vi "FetchCalibration.vi"(8 "error in (no error)":errorcluster, 10 "instruments":string[](array[string]), 11 "ByteGSAPIBase in":refnum<class "ByteGSAPIBase.lvclass">) -> (0 "error out":errorcluster, 2 "instruments":T1[](array[typedef]), 3 "ByteGSAPIBase out":refnum<class "ByteGSAPIBase.lvclass">)   [LabVIEW 2019, in "ByteGSWebAPI.lvlib" / "ByteGSAPIBase.lvclass"]
doc: "Obtain instruments calibrations based on the Instrument Slug"
uses:
  ByteGSAPIBase.lvclass
  Converted_Slug_Cluster.ctl
  <vilib>/Bytelabs/ByteREST/ByteRESTClass/ByteRESTBase/HTTP/Status_Code.ctl
  JSON_Slug_Cluster.ctl
  ByteGSAPIBase.lvclass/ByteGSAPIBase.ctl
  <vilib>/Bytelabs/ByteREST/ByteRESTClass/ByteRESTBase/RESTBase.lvclass
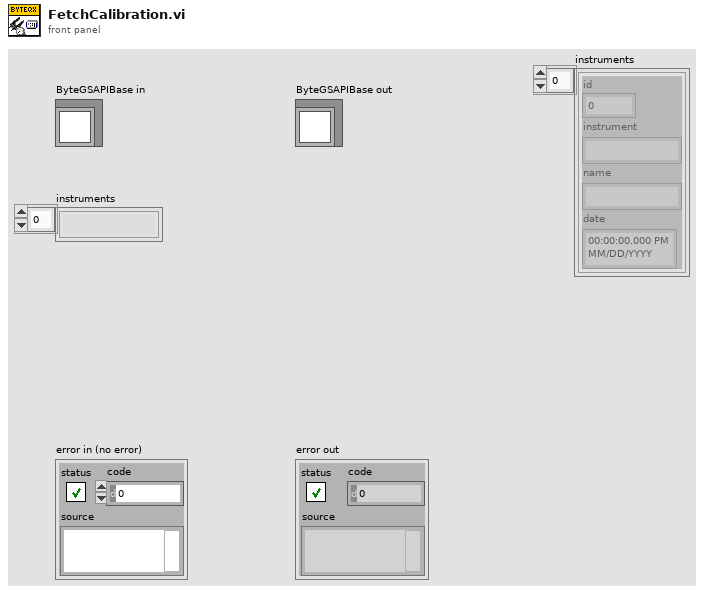
[diagram p1: front panel]
types:
  T1 = typedef "ByteGSWebAPI.lvlib/ByteGSAPIBase.lvclass/Converted_Slug_Cluster.ctl" = cluster{"id":u32, "instrument":string, "name":string, "date":timestamp}
  T2 = typedef "ByteGSWebAPI.lvlib/ByteGSAPIBase.lvclass/JSON_Slug_Cluster.ctl" = cluster{"id":u32, "instrument":string, "name":string, "data":string}
  T3 = typedef "ByteREST.lvlib/RESTBase.lvclass/Status_Code.ctl" = u16
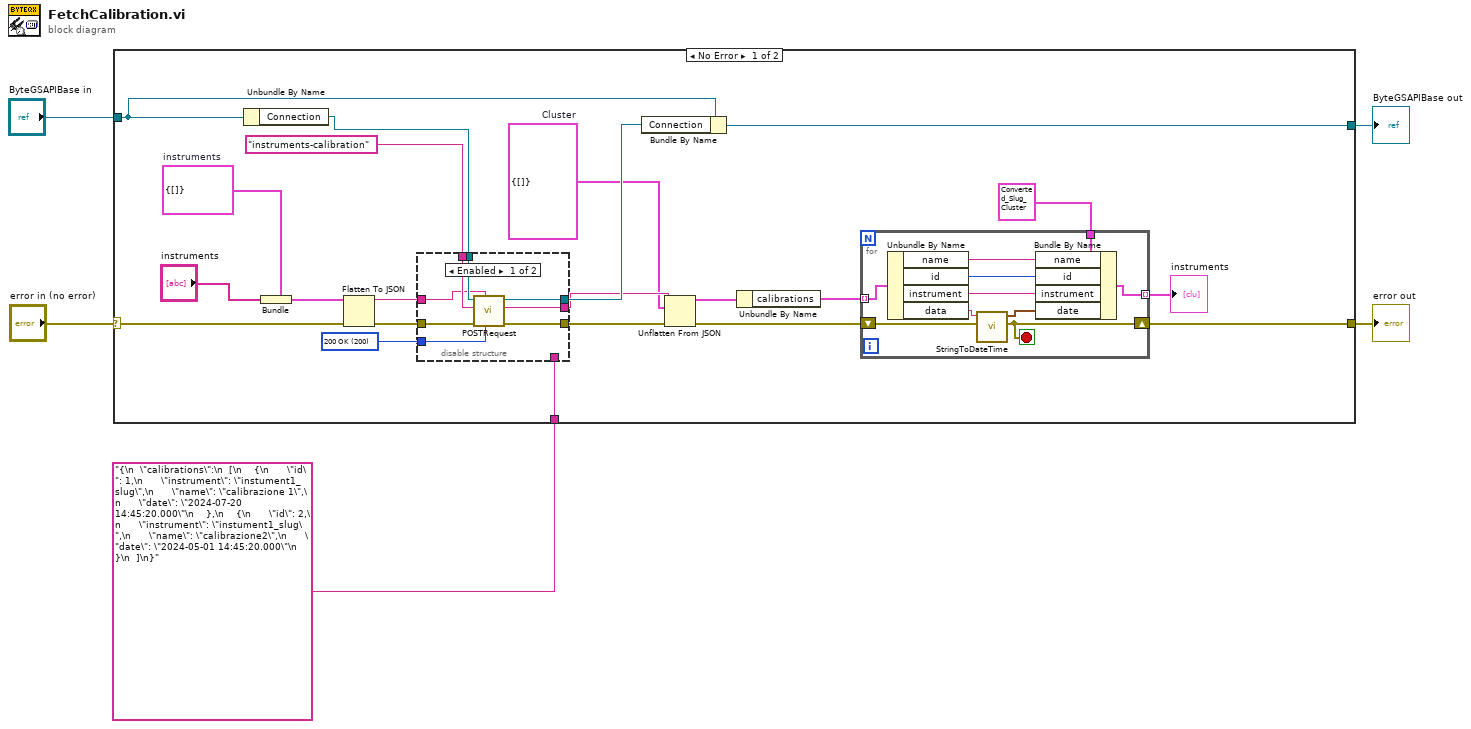
[diagram p0: block diagram]
diagram:
  n1 = case shown="No Error" "error in (no error)" {
    selector: "error in (no error)" -> [w22 w48]
    tunnel: [w14 w48] -> w4
    tunnel: [w25 w47] -> w2
    tunnel: "ByteGSAPIBase in" -> [w27 w47]
    tunnel: "{\n  \"calibrations\":\n  [\n    {\n      \"id\": 1,\n      \"instrument\": \"instument1_slug\",\n      \"name\": \"calibrazione 1\",\n      \"date\": \"2024-07-20 14:45:20.000\"\n    },\n    {\n      \"id\": 2,\n      \"instrument\": \"instument1_slug\",\n      \"name\": \"calibrazione2\",\n      \"date\": \"2024-05-01 14:45:20.000\"\n    }\n  ]\n}" ("Body") -> [w10 _]
    frame No Error {
      w7 = cluster{"calibrations":T2[]} {"calibrations"=[]}  # Cluster
      w13 = cluster{"instruments":string[]} {"instruments"=[]}  # instruments
      w19 = T3 200 items=["200 OK"=200, "201 Created"=201, "400 Bad Request"=400, "401 Unauthorized"=401, "403 Forbidden"=403, "404 Not Found"=404, "405 Method Not Allowed"=405, "406 Not Acceptable"=406, "500 Internal Server Error"=500] ("expected response")
      n2 = Unbundle By Name(w27) -> ("Connection"=w26:refnum<class "RESTBase.lvclass">)
      n3 = Bundle(cluster=w13, "instruments"="instruments") -> (w11:cluster{"instruments":string[]})
      n4 = Flatten To JSON(anything=w11, error in (no error)=w22) -> (JSON string=w17:string, 11:w18:errorcluster)  [unwired: 1 in]
      n5 = disable-structure shown="Enabled" {
        disable-tunnel: w26 -> [w45 _]
        disable-tunnel: [w44 _] -> w24
        disable-tunnel: "instruments-calibration" ("Request") -> [w43 _]
        disable-tunnel: [w42 w46] -> w21
        disable-tunnel: [w41 _] -> w20
        disable-tunnel: w19 -> [w40 _]
        disable-tunnel: w18 -> [w39 _]
        disable-tunnel: w17 -> [w38 _]
        disable-tunnel: w10 -> [_ w46]
        frame Enabled {
          n6 = call-dynamic "POSTRequest.vi"("expected response"=w40, "Body in"=w38, "error in (no error)"=w39, "Request"=w43, "ByteRESTBase in"=w45) -> ("error out"=w41:errorcluster, "Body"=w42:string, "ByteRESTBase out"=w44:refnum<class "RESTBase.lvclass">)  [unwired: 3 in, 1 out]
        }
        frame Disabled {
        }
      }
      n7 = Bundle By Name(cluster=w27, "Connection"=w24) -> (w25:refnum<class "ByteGSAPIBase.lvclass">)
      n8 = Unflatten From JSON(JSON string=w21, type and defaults=w7, error in (no error)=w20) -> (value=w16:cluster{"calibrations":T2[]}, error out=w15:errorcluster)  [unwired: 4 in]
      n9 = Unbundle By Name(w16) -> ("calibrations"=w9:T2[])
      n10 = for {
        tunnel: w9 -> [w37] mode=indexing
        tunnel: [w32] -> w8 mode=indexing
        tunnel: T1 {"id"=0, "instrument"="", "name"="", "date"=timestamp(0 s since 1904-01-01)} ("Converted_Slug_Cluster") -> [w29]
        shift-right: [w30] -> w14
        shift-left: w15 -> [w31]
        stop <- w30 stop-if-true
        n11 = Unbundle By Name(w37) -> ("name"=w28:string, "id"=w36:u32, "instrument"=w33:string, "data"=w35:string)
        n12 = call "StringToDateTime.vi"("error in (no error)"=w31, "datetime string"=w35) -> ("error out"=w30:errorcluster, "timestamp"=w34:timestamp)  [unwired: 8 in]
        n13 = Bundle By Name(cluster=w29, "name"=w28, "id"=w36, "instrument"=w33, "date"=w34) -> (w32:T1)
      }
      "instruments" <- w8
    }
    frame Error {
    }
  }
  "error out" <- w4
  "ByteGSAPIBase out" <- w2
